vi "HomeWork3.vi"(3 "Voltage":dbl) -> (0 "Mahtuvus ( F )":dbl, 1 "Takistus (Oom)":dbl, 2 "RC":dbl, 5 "Time":dbl, 6 "TimeStep":dbl, 7 "Time array":dbl[][](array[numeric]), 8 "Waveform Graph":cluster{dbl, "Ajasamm ( 0.01 sec)":dbl, dbl[]}[](graph), 9 "Discharging waveform":waveform(dbl), 10 "Charging waveform":waveform(dbl))   [LabVIEW 2018]
doc: "This Sub_Vi calculates the time behavior of the capacitor charging and discharging (voltage variation on capacitor C - sub-VI outputs (Waveforms) Charging and Discharging) of a predetermined resistor (input R, kO), capacitor (input C, µF) and charging voltage (input Umax, V )."
panel:
  out "Waveform Charging + Discharging":cluster{dbl, dbl}[](graph)
  out "DisCharging":dbl
  out "Exp(x)Charging":dbl
  out "Charging":dbl
  out "Exp(x)Discharging":dbl
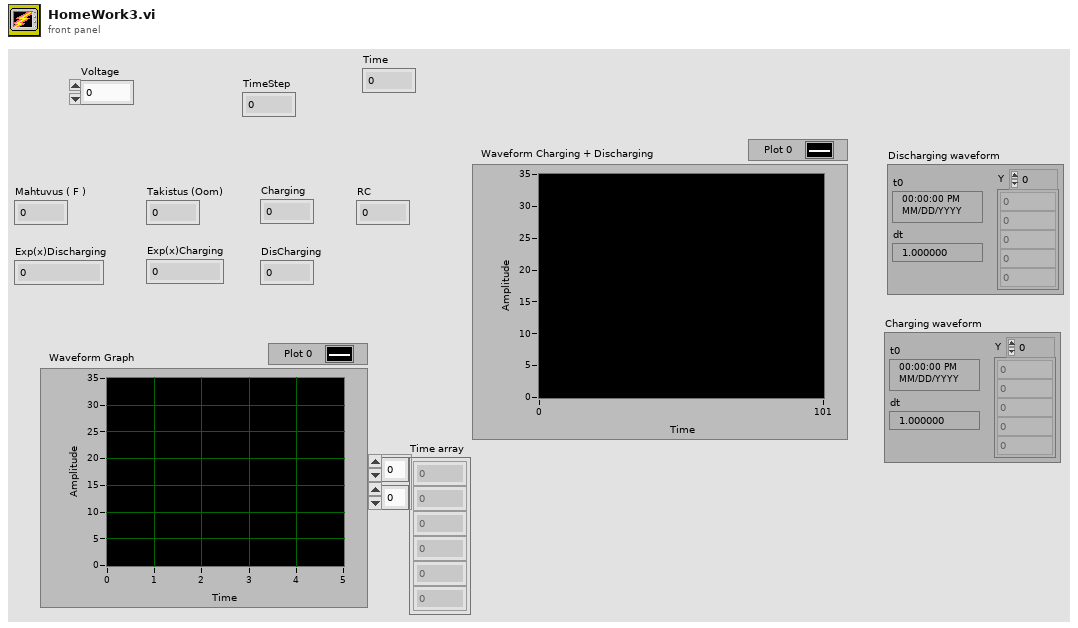
[diagram p1: front panel]
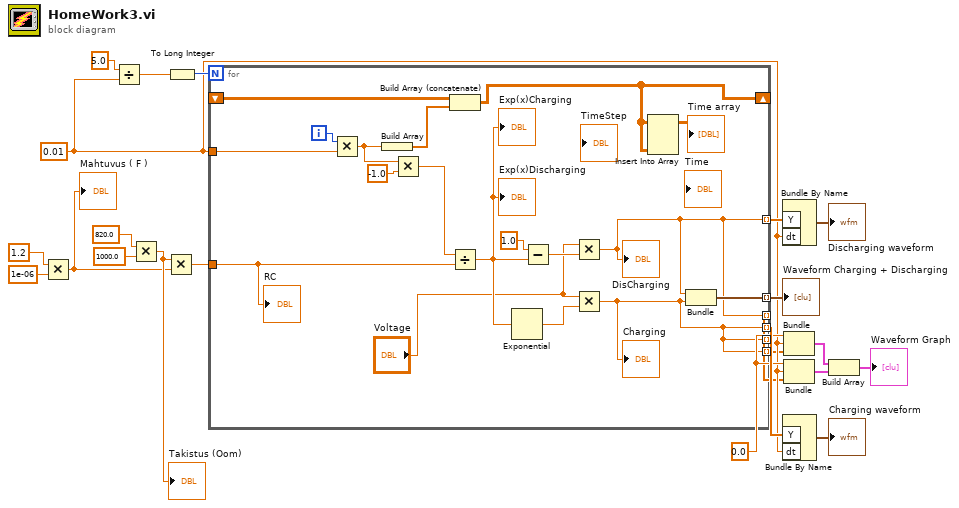
[diagram p0: block diagram]
diagram:
  w7 = 0.0
  w6 = 0.01 ("Ajasamm ( 0.01 sec)")
  n1 = Multiply(x=1.2 ("Mahtuvus ( 1.2 uF )"), y=1e-06) -> (x*y=w13:dbl)
  "Mahtuvus ( F )" <- w13
  n2 = Divide(x=5.0, y=w6) -> (x/y=w15:dbl)
  n3 = Multiply(x=820.0 ("Takistus (kOom)"), y=1000.0) -> (x*y=w14:dbl)
  "Takistus (Oom)" <- w14
  n4 = Multiply(x=w14, y=w13) -> (x*y=w8:dbl)
  n5 = To Long Integer(number=w15) -> (32bit integer=w16:i32)
  n6 = for {
    N: w16 -> [_]
    tunnel: [w36] -> w22 mode=indexing
    tunnel: [w27] -> _ mode=indexing
    tunnel: [w26] -> w20 mode=indexing
    tunnel: [w27] -> w19 mode=indexing
    tunnel: w6 -> [w32]
    shift-right: [w25] -> _
    shift-left: _ -> [w30]
    tunnel: w8 -> [w28]
    tunnel: [w27] -> w5 mode=indexing
    tunnel: [w26] -> w4 mode=indexing
    i -> [w35]
    n7 = Multiply(x=w35, y=w32) -> (x*y=w31:dbl)
    n8 = Build Array(w31) -> (w29:dbl[])
    n9 = Multiply(x=w31, y=-1.0) -> (x*y=w33:dbl)
    n10 = Build Array (concatenate)(w30, w29) -> (w25:dbl[][])
    n11 = Divide(x=w33, y=w28) -> (x/y=w37:dbl)
    "Exp(x)Discharging" <- w37
    "Exp(x)Charging" <- w37
    n12 = Exponential(1:w37) -> (0:w40:dbl)
    n13 = Subtract(x=1.0, y=w37) -> (x-y=w38:dbl)
    n14 = Multiply(x="Voltage", y=w38) -> (x*y=w26:dbl)
    "DisCharging" <- w26
    n15 = Multiply(x="Voltage", y=w40) -> (x*y=w27:dbl)
    "Charging" <- w27
    n16 = Insert Into Array(array=w25, new element=w25) -> (→"Time array":dbl[][])  [unwired: 2 in]
    n17 = Bundle(w26, w27) -> (w36:cluster{dbl, dbl})  [unwired: 1 in]
    "RC" <- w28
  }
  "Waveform Charging + Discharging" <- w22
  n18 = Bundle By Name("Y"=w20, "dt"=w6) -> (→"Discharging waveform":waveform(dbl))  [unwired: 1 in]
  n19 = Bundle By Name("Y"=w19, "dt"=w6) -> (→"Charging waveform":waveform(dbl))  [unwired: 1 in]
  n20 = Bundle(w7, "Ajasamm ( 0.01 sec)"=w6, w5) -> (w3:cluster{dbl, "Ajasamm ( 0.01 sec)":dbl, dbl[]})  [unwired: 1 in]
  n21 = Bundle(w7, "Ajasamm ( 0.01 sec)"=w6, w4) -> (w2:cluster{dbl, "Ajasamm ( 0.01 sec)":dbl, dbl[]})  [unwired: 1 in]
  n22 = Build Array(w3, w2) -> (→"Waveform Graph":cluster{dbl, "Ajasamm ( 0.01 sec)":dbl, dbl[]}[])
